vi "set num to enum.vi"(1 "Numeric in":u8) -> (0 "Numeric out":T1)   [LabVIEW 2021]
uses:
  pulse_tx_vis/CTL/mode_type.ctl
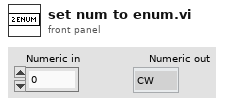
[diagram p1: front panel]
types:
  T1 = typedef "mode_type.ctl" = enum8{"CW", "from memory 1", "NC - cw", "LFM", "BPSK", "QPSK"}
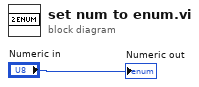
[diagram p0: block diagram]
diagram:
  "Numeric out" <- "Numeric in"
